vi "CreateReportDirectory.vi"(5 "error in (no error)":errorcluster) -> (14 "ReportDirectory":path, 16 "ProjectFile":path, 19 "error out":errorcluster)   [LabVIEW 2020]
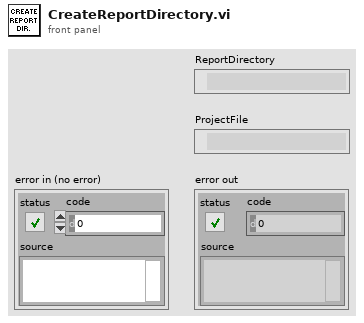
[diagram p1: front panel]
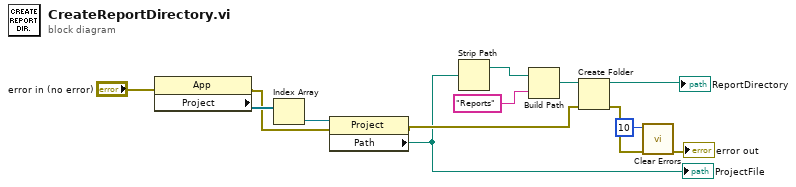
[diagram p0: block diagram]
diagram:
  n1 = property class="App"(error in="error in (no error)") -> (error out=w7:errorcluster, "Project"=w13:refnum<vi>[])  [unwired: 1 in, 1 out]
  n2 = Index Array(array=w13) -> (element=w12:refnum<vi>)  [unwired: 1 in]
  n3 = property class="Project"(reference=w12, error in=w7) -> (error out=w8:errorcluster, "Path"=w5:path)  [unwired: 1 out]
  "ProjectFile" <- w5
  n4 = Strip Path(path=w5) -> (stripped path=w11:path)  [unwired: 1 out]
  n5 = Build Path(base path=w11, name or relative path="Reports") -> (appended path=w9:path)
  n6 = Create Folder(path (use dialog)=w9, error in=w8) -> (created path=→"ReportDirectory":path, error out=w3:errorcluster)  [unwired: 1 in, 1 out]
  n7 = call <vilib>:"Clear Errors.vi"("error in (no error)"=w3, "specific error code to clear (0: all)"=10 ("error code (0)")) -> ("error out"=→"error out":errorcluster)  [unwired: 4 in, 1 out]
